vi "Demo_Get shift.vi"(8 "error in (no error)":errorcluster, 11 "Shift Time Details":T1={"1Start"=timestamp(5400 s since 1904-01-01), "1End"=timestamp(34200 s since 1904-01-01), "2Start"=timestamp(34200 s since 1904-01-01), "3Start"=timestamp(63000 s since 1904-01-01), "2End"=timestamp(63000 s since 1904-01-01), "3End"=timestamp(5400 s since 1904-01-01)} {"3End" format="%<%H:%M:%S>T"; "2End" format="%<%H:%M:%S>T"; "3Start" format="%<%H:%M:%S>T"; "2Start" format="%<%H:%M:%S>T"; "1End" format="%<%H:%M:%S>T"; "1Start" format="%<%H:%M:%S>T"}) -> (0 "error out":errorcluster, 2 "Shift":i32, 3 "Date":string)   [LabVIEW 2017]
panel:
  # "Start Time"
  # "End Time"
  # "Shift-1"
  # "Shift-2"
  # "Shift-3"
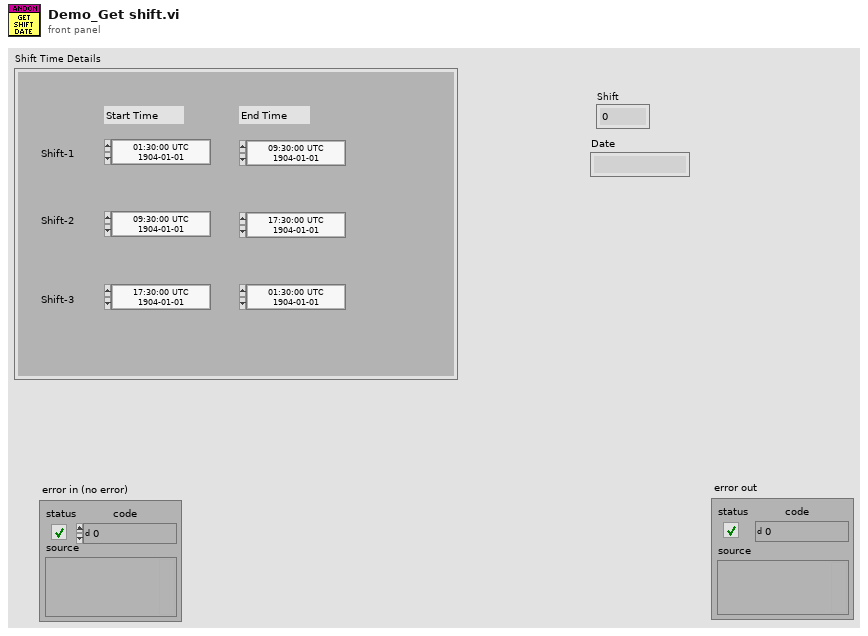
[diagram p1: front panel]
types:
  T1 = cluster{"1Start":timestamp, "1End":timestamp, "2Start":timestamp, "3Start":timestamp, "2End":timestamp, "3End":timestamp}
  T2 = typedef "LVDateTimeRec.ctl" = cluster{"fractional second":dbl, "second":i32, "minute":i32, "hour":i32, "day of month":i32, "month":i32, "year":i32, "day of week":i32, "day of year":i32, "DST":i32}
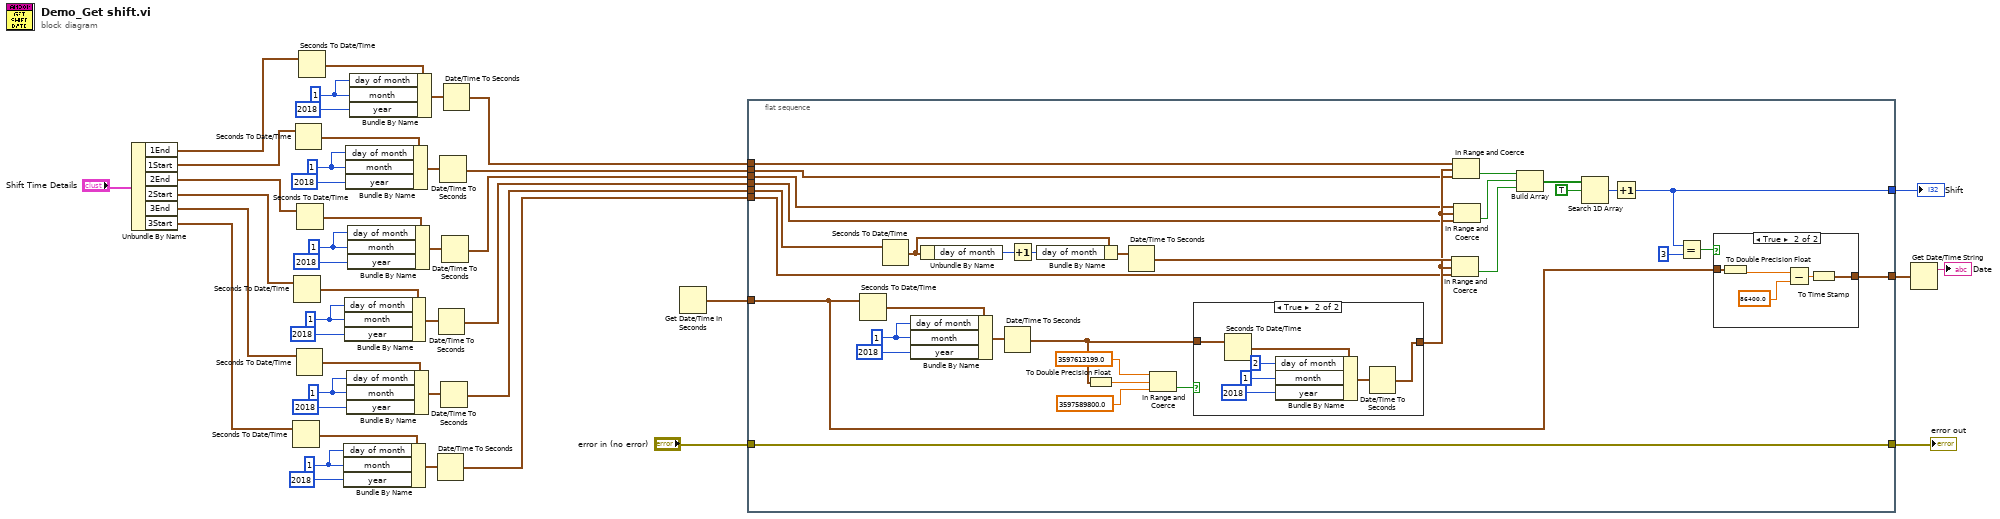
[diagram p0: block diagram]
diagram:
  w13 = 1 ("day of month")
  w19 = 1 ("day of month")
  w27 = 1 ("day of month")
  w20 = 1 ("day of month")
  w31 = 1 ("day of month")
  w39 = 1 ("day of month")
  n1 = Unbundle By Name("Shift Time Details") -> ("1End"=w35:timestamp, "1Start"=w30:timestamp, "2End"=w12:timestamp, "2Start"=w11:timestamp, "3End"=w6:timestamp, "3Start"=w5:timestamp)
  n2 = Seconds To Date/Time(time stamp (now)=w5) -> (date time rec=w4:T2)  [unwired: 1 in]
  n3 = Seconds To Date/Time(time stamp (now)=w11) -> (date time rec=w26:T2)  [unwired: 1 in]
  n4 = Seconds To Date/Time(time stamp (now)=w30) -> (date time rec=w32:T2)  [unwired: 1 in]
  n5 = Seconds To Date/Time(time stamp (now)=w6) -> (date time rec=w18:T2)  [unwired: 1 in]
  n6 = Seconds To Date/Time(time stamp (now)=w12) -> (date time rec=w21:T2)  [unwired: 1 in]
  n7 = Seconds To Date/Time(time stamp (now)=w35) -> (date time rec=w38:T2)  [unwired: 1 in]
  n8 = Bundle By Name(cluster=w4, "day of month"=w13, "month"=w13, "year"=2018) -> (w15:T2)
  n9 = Bundle By Name(cluster=w26, "day of month"=w27, "month"=w27, "year"=2018) -> (w24:T2)
  n10 = Bundle By Name(cluster=w32, "day of month"=w31, "month"=w31, "year"=2018) -> (w34:T2)
  n11 = Bundle By Name(cluster=w18, "day of month"=w19, "month"=w19, "year"=2018) -> (w16:T2)
  n12 = Bundle By Name(cluster=w21, "day of month"=w20, "month"=w20, "year"=2018) -> (w23:T2)
  n13 = Bundle By Name(cluster=w38, "day of month"=w39, "month"=w39, "year"=2018) -> (w36:T2)
  n14 = Date/Time To Seconds(2:w15) -> (0:w7:timestamp)  [unwired: 1 in]
  n15 = Date/Time To Seconds(2:w24) -> (0:w9:timestamp)  [unwired: 1 in]
  n16 = Date/Time To Seconds(2:w34) -> (0:w28:timestamp)  [unwired: 1 in]
  n17 = Date/Time To Seconds(2:w16) -> (0:w8:timestamp)  [unwired: 1 in]
  n18 = Date/Time To Seconds(2:w23) -> (0:w10:timestamp)  [unwired: 1 in]
  n19 = Date/Time To Seconds(2:w36) -> (0:w29:timestamp)  [unwired: 1 in]
  n20 = Get Date/Time In Seconds() -> (seconds since 1Jan1904=w1:timestamp)
  n21 = flat-sequence {
    tunnel: [w46] -> w43
    tunnel: "error in (no error)" -> [w56]
    tunnel: [w56] -> w41
    tunnel: w1 -> [w48]
    tunnel: w29 -> [w55]
    tunnel: w28 -> [w54]
    tunnel: w10 -> [w53]
    tunnel: w9 -> [w52]
    tunnel: w8 -> [w51]
    tunnel: w7 -> [w50]
    tunnel: [w47] -> w3
    frame #0 {
      w60 = 1 ("day of month")
      n22 = Seconds To Date/Time(time stamp (now)=w48) -> (date time rec=w49:T2)  [unwired: 1 in]
      n23 = Seconds To Date/Time(time stamp (now)=w51) -> (date time rec=w75:T2)  [unwired: 1 in]
      n24 = Bundle By Name(cluster=w49, "day of month"=w60, "month"=w60, "year"=2018) -> (w65:T2)
      n25 = Unbundle By Name(w75) -> ("day of month"=w73:i32)
      n26 = Date/Time To Seconds(2:w65) -> (0:w58:timestamp)  [unwired: 1 in]
      n27 = Increment(x=w73) -> (x+1=w74:i32)
      n28 = Bundle By Name(cluster=w75, "day of month"=w74) -> (w76:T2)
      n29 = To Double Precision Float(number=w58) -> (double precision float=w61:dbl)
      n30 = Date/Time To Seconds(2:w76) -> (0:w72:timestamp)  [unwired: 1 in]
      n31 = In Range and Coerce(upper limit=3597613199.0 ("double precision float 2"), x=w61, lower limit=3597589800.0 ("double precision float")) -> (In Range?=w59:bool)  [unwired: 1 out]
      n32 = case shown="True" w59 {
        tunnel: w58 -> [w83 w86]
        tunnel: [w83 w85] -> w57
        frame False {
        }
        frame True {
          n33 = Seconds To Date/Time(time stamp (now)=w86) -> (date time rec=w88:T2)  [unwired: 1 in]
          n34 = Bundle By Name(cluster=w88, "day of month"=2, "month"=1 ("day of month"), "year"=2018) -> (w90:T2)
          n35 = Date/Time To Seconds(2:w90) -> (0:w85:timestamp)  [unwired: 1 in]
        }
      }
      n36 = In Range and Coerce(upper limit=w72, x=w57, lower limit=w50) -> (In Range?=w69:bool)  [unwired: 1 out]
      n37 = In Range and Coerce(upper limit=w55, x=w57, lower limit=w54) -> (In Range?=w71:bool)  [unwired: 1 out]
      n38 = In Range and Coerce(upper limit=w53, x=w57, lower limit=w52) -> (In Range?=w70:bool)  [unwired: 1 out]
      n39 = Build Array(w71, w70, w69) -> (w68:bool[])
      n40 = Search 1D Array(1D array=w68, element=TRUE) -> (index of element=w66:i32)  [unwired: 1 in]
      n41 = Increment(x=w66) -> (x+1=w46:i32)
      n42 = Equal?(x=w46, y=3) -> (x = y?=w44:bool)
      n43 = case shown="True" w44 {
        tunnel: w48 -> [w77 w79]
        tunnel: [w77 w78] -> w47
        frame False {
        }
        frame True {
          n44 = To Double Precision Float(number=w79) -> (double precision float=w81:dbl)
          n45 = Subtract(x=w81, y=86400.0) -> (x-y=w82:dbl)
          n46 = To Time Stamp(1:w82) -> (0:w78:timestamp)
        }
      }
    }
  }
  n47 = Get Date/Time String(seconds (now)=w3) -> (date string=→"Date":string)  [unwired: 2 in, 1 out]
  "Shift" <- w43
  "error out" <- w41
